vi "InAs-GaAs superlattice-111227a.vi"() -> ()   [LabVIEW 2011]
panel:
  out "step number  5":i32
  in  "Number of \nGrowth Steps 5":i32=10
  out "step number  4":i32
  in  "Number of \nGrowth Steps 4":i32=10
  out "step number  3":i32
  in  "Number of \nGrowth Steps 3":i32=10
  out "step number  2":i32
  in  "Number of \nGrowth Steps 2":i32=10
  in  "Ga Flow 1":dbl=5.49
  in  "Indium Flow":dbl=45.0
  in  "Number of \nGrowth Steps":i32=10
  out "step number":i32
  in  "As_Gas Flow":dbl=3.4
  in  "Manifold H2 Flow":dbl=730.0
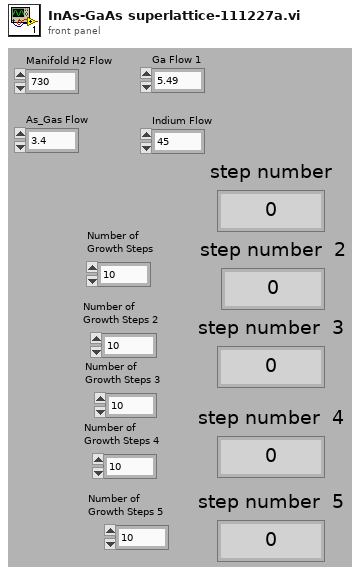
[diagram p1: front panel]
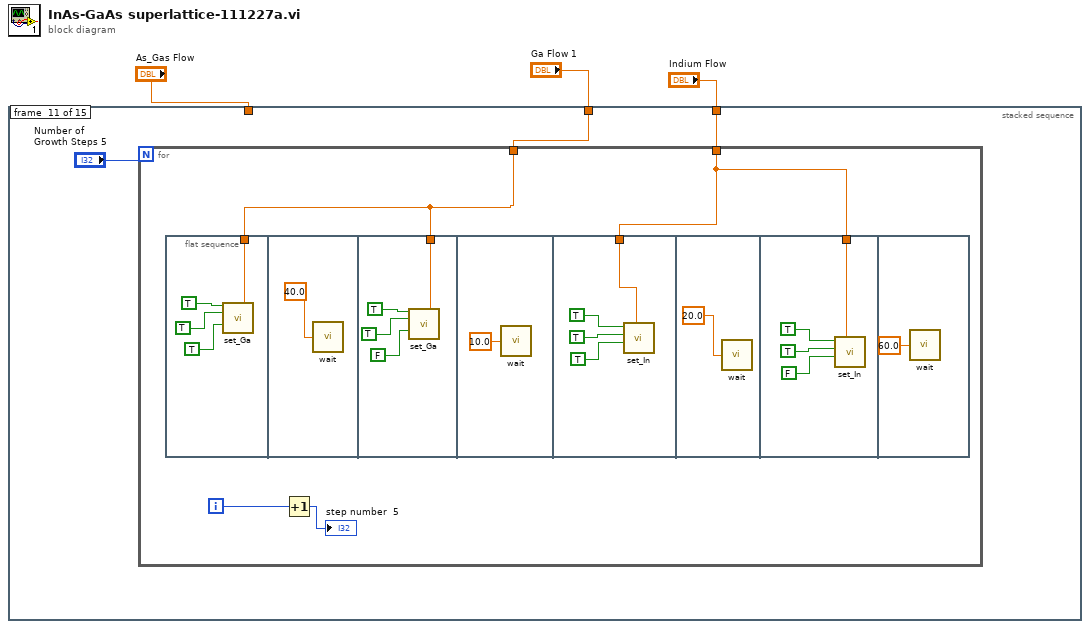
[diagram p0: block diagram]
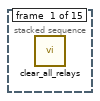
[diagram p2: hidden frame]
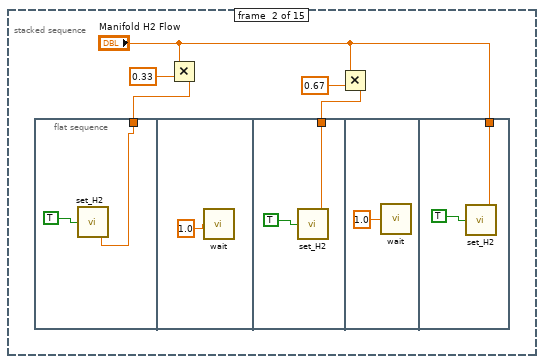
[diagram p3: hidden frame]
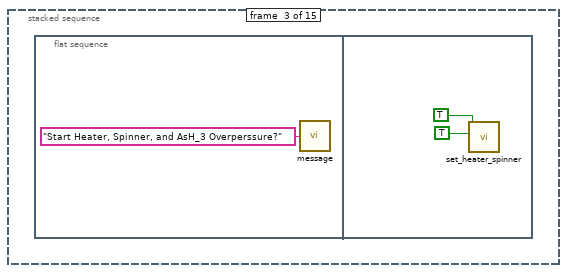
[diagram p4: hidden frame]
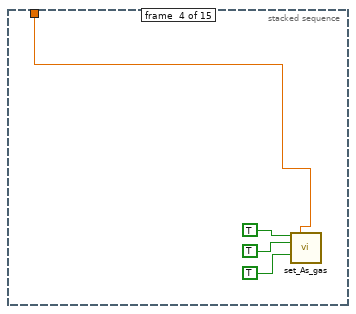
[diagram p5: hidden frame]
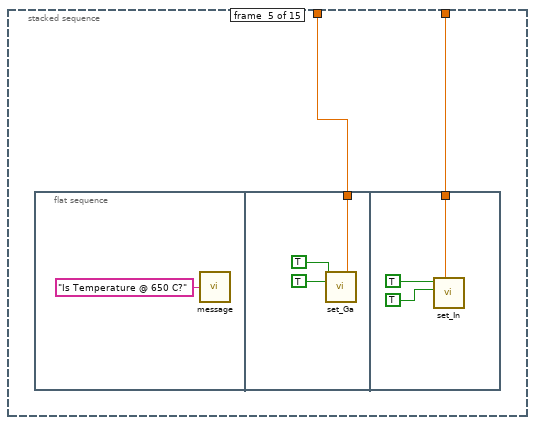
[diagram p6: hidden frame]
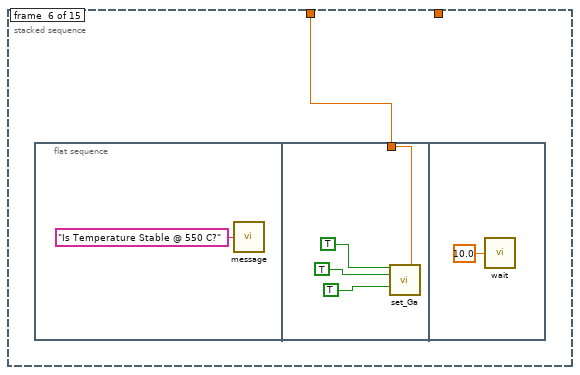
[diagram p7: hidden frame]
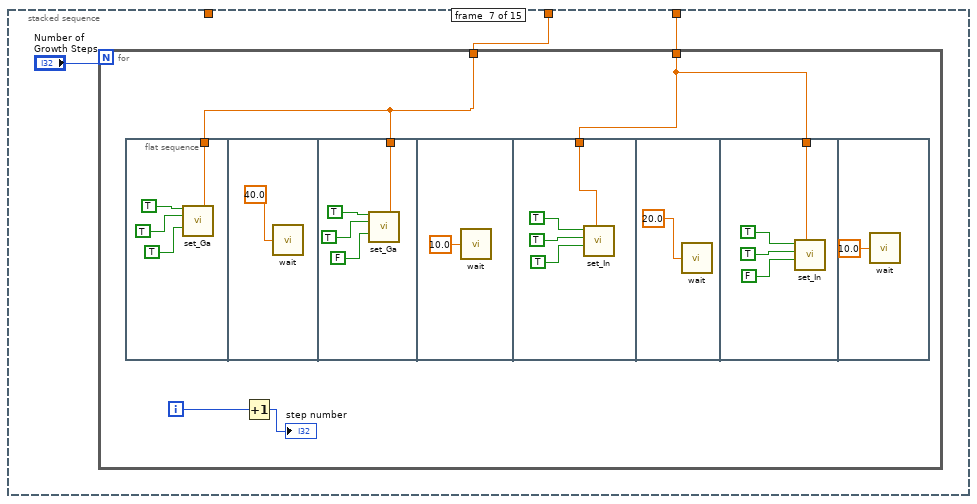
[diagram p8: hidden frame]
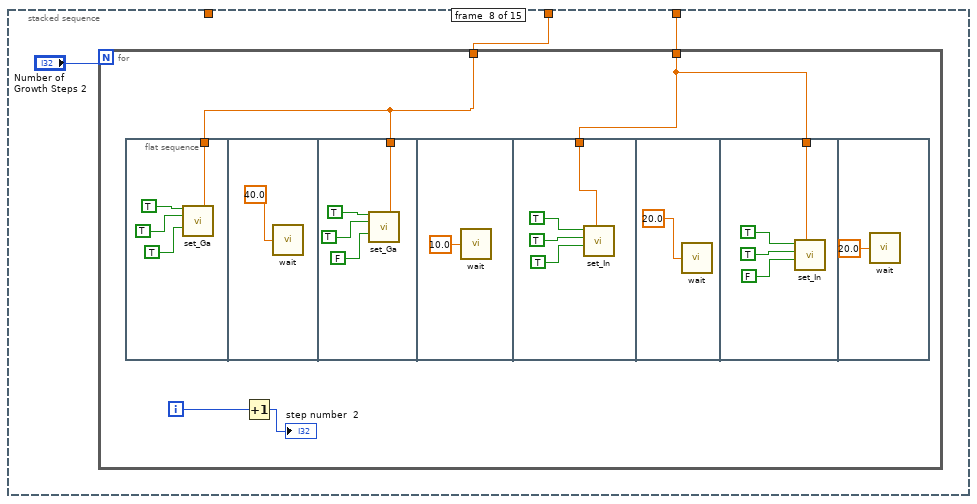
[diagram p9: hidden frame]
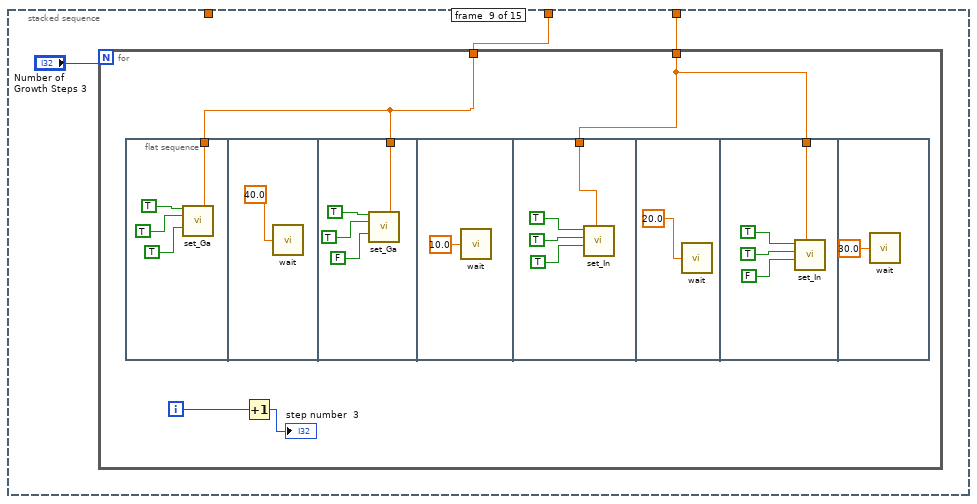
[diagram p10: hidden frame]
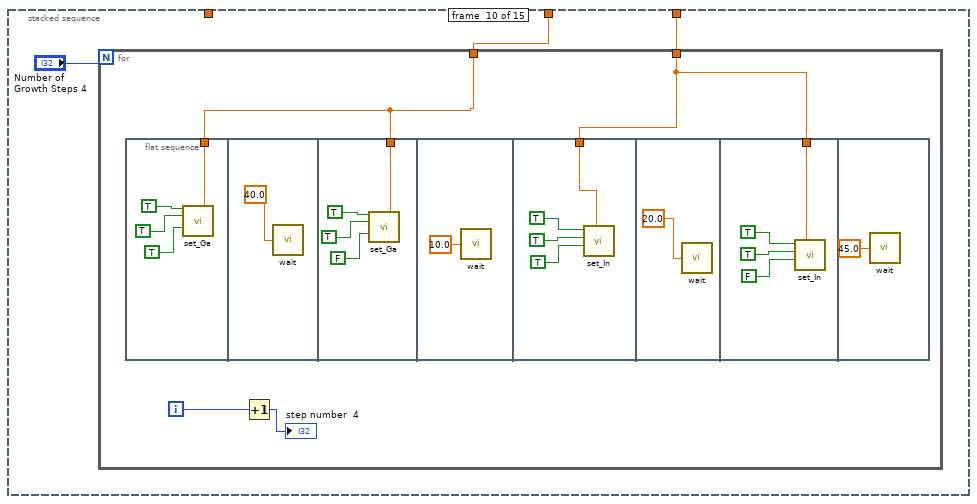
[diagram p11: hidden frame]
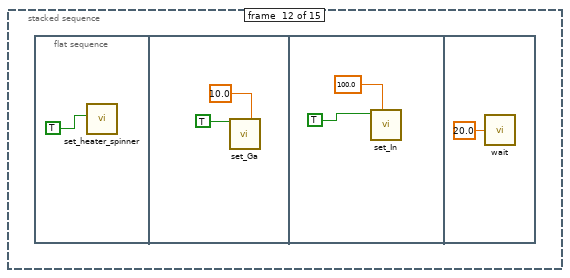
[diagram p12: hidden frame]
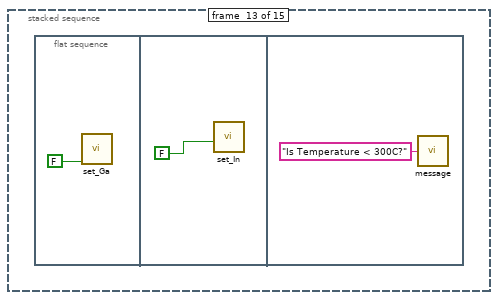
[diagram p13: hidden frame]
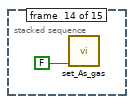
[diagram p14: hidden frame]
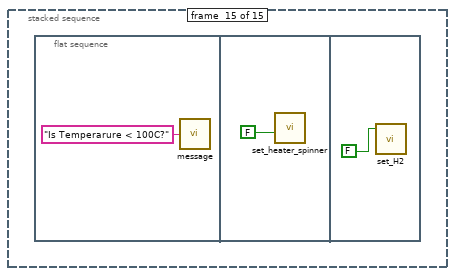
[diagram p15: hidden frame]
diagram:
  n1 = stacked-sequence {
    tunnel: "Ga Flow 1" -> [_ _ _ _ w25 w33 w41 w68 w95 w122 w149 _ _ _ _]
    tunnel: "As_Gas Flow" -> [_ _ _ w20 _ _ _ _ _ _ _ _ _ _ _]
    tunnel: "Indium Flow" -> [_ _ _ _ w24 _ w40 w67 w94 w121 w148 _ _ _ _]
    frame #0 {
      n2 = call "clear_all_relays.vi"() -> ()  [unwired: 2 out]
    }
    frame #1 {
      n3 = flat-sequence {
        tunnel: w8 -> [w9]
        tunnel: w6 -> [w12]
        tunnel: "Manifold H2 Flow" -> [w15]
        frame #0 {
          n4 = call "set_H2.vi"("Manifold H2 Flow"=w9, "H2 Active"=TRUE) -> ()  [unwired: 2 in, 2 out]
        }
        frame #1 {
          n5 = call "wait.vi"("Wait (s)"=1.0) -> ()  [unwired: 1 out]
        }
        frame #2 {
          n6 = call "set_H2.vi"("Manifold H2 Flow"=w12, "H2 Active"=TRUE) -> ()  [unwired: 2 in, 2 out]
        }
        frame #3 {
          n7 = call "wait.vi"("Wait (s)"=1.0) -> ()  [unwired: 1 out]
        }
        frame #4 {
          n8 = call "set_H2.vi"("Manifold H2 Flow"=w15, "H2 Active"=TRUE) -> ()  [unwired: 2 in, 2 out]
        }
      }
      n9 = Multiply(x="Manifold H2 Flow", y=0.33) -> (x*y=w8:dbl)
      n10 = Multiply(x="Manifold H2 Flow", y=0.67) -> (x*y=w6:dbl)
    }
    frame #2 {
      n11 = flat-sequence {
        frame #0 {
          n12 = call "message.vi"("message"="Start Heater, Spinner, and AsH_3 Overperssure?") -> ()
        }
        frame #1 {
          n13 = call "set_heater_spinner.vi"("Spinner"=TRUE, "Heater"=TRUE) -> ()  [unwired: 1 in, 7 out]
        }
      }
    }
    frame #3 {
      n14 = call "set_As_gas.vi"("As_Gas Active"=TRUE, "As_Gas Flow"=w20, "As_Gas In"=TRUE, "As_Gas Run"=TRUE) -> ()  [unwired: 2 in, 10 out]
    }
    frame #4 {
      n15 = flat-sequence {
        tunnel: w25 -> [w27]
        tunnel: w24 -> [w30]
        frame #0 {
          n16 = call "message.vi"("message"="Is Temperature @ 650 C?") -> ()
        }
        frame #1 {
          n17 = call "set_Ga.vi"("Ga Active"=TRUE, "Ga Flow 1"=w27, "Ga Bubbler"=TRUE) -> ()  [unwired: 5 in, 8 out]
        }
        frame #2 {
          n18 = call "set_In.vi"("Indium Flow"=w30, "In Bubbler"=TRUE ("Ga Bubbler"), "In Active"=TRUE ("Ga Active")) -> ()  [unwired: 2 in, 5 out]
        }
      }
    }
    frame #5 {
      n19 = flat-sequence {
        tunnel: w33 -> [w35]
        frame #0 {
          n20 = call "message.vi"("message"="Is Temperature Stable @ 550 C?") -> ()
        }
        frame #1 {
          n21 = call "set_Ga.vi"("Ga Active"=TRUE ("P_Gas Active"), "Ga Flow 1"=w35, "Ga Bubbler"=TRUE ("P_Gas In"), "Ga Run"=TRUE ("P_Gas Run")) -> ()  [unwired: 4 in, 8 out]
        }
        frame #2 {
          n22 = call "wait.vi"("Wait (s)"=10.0) -> ()  [unwired: 1 out]
        }
      }
    }
    frame #6 {
      n23 = for {
        N: "Number of \nGrowth Steps" -> [_]
        tunnel: w41 -> [w44]
        tunnel: w40 -> [w43]
        i -> [w45]
        n24 = flat-sequence {
          tunnel: w44 -> [w47]
          tunnel: w44 -> [w52]
          tunnel: w43 -> [w57]
          tunnel: w43 -> [w62]
          frame #0 {
            n25 = call "set_Ga.vi"("Ga Active"=TRUE ("P_Gas Active"), "Ga Flow 1"=w47, "Ga Bubbler"=TRUE ("P_Gas In"), "Ga Run"=TRUE ("P_Gas Run")) -> ()  [unwired: 4 in, 8 out]
          }
          frame #1 {
            n26 = call "wait.vi"("Wait (s)"=40.0) -> ()  [unwired: 1 out]
          }
          frame #2 {
            n27 = call "set_Ga.vi"("Ga Active"=TRUE ("P_Gas Active"), "Ga Flow 1"=w52, "Ga Bubbler"=TRUE ("P_Gas In"), "Ga Run"=FALSE ("P_Gas Run")) -> ()  [unwired: 4 in, 8 out]
          }
          frame #3 {
            n28 = call "wait.vi"("Wait (s)"=10.0) -> ()  [unwired: 1 out]
          }
          frame #4 {
            n29 = call "set_In.vi"("Indium Flow"=w57, "In Run"=TRUE ("P_Gas Run"), "In Bubbler"=TRUE ("P_Gas In"), "In Active"=TRUE ("P_Gas Active")) -> ()  [unwired: 1 in, 5 out]
          }
          frame #5 {
            n30 = call "wait.vi"("Wait (s)"=20.0) -> ()  [unwired: 1 out]
          }
          frame #6 {
            n31 = call "set_In.vi"("Indium Flow"=w62, "In Run"=FALSE ("P_Gas Run"), "In Bubbler"=TRUE ("P_Gas In"), "In Active"=TRUE ("P_Gas Active")) -> ()  [unwired: 1 in, 5 out]
          }
          frame #7 {
            n32 = call "wait.vi"("Wait (s)"=10.0) -> ()  [unwired: 1 out]
          }
        }
        n33 = Increment(x=w45) -> (x+1=→"step number":i32)
      }
    }
    frame #7 {
      n34 = for {
        N: "Number of \nGrowth Steps 2" -> [_]
        tunnel: w68 -> [w71]
        tunnel: w67 -> [w70]
        i -> [w72]
        n35 = flat-sequence {
          tunnel: w71 -> [w74]
          tunnel: w71 -> [w79]
          tunnel: w70 -> [w84]
          tunnel: w70 -> [w89]
          frame #0 {
            n36 = call "set_Ga.vi"("Ga Active"=TRUE ("P_Gas Active"), "Ga Flow 1"=w74, "Ga Bubbler"=TRUE ("P_Gas In"), "Ga Run"=TRUE ("P_Gas Run")) -> ()  [unwired: 4 in, 8 out]
          }
          frame #1 {
            n37 = call "wait.vi"("Wait (s)"=40.0) -> ()  [unwired: 1 out]
          }
          frame #2 {
            n38 = call "set_Ga.vi"("Ga Active"=TRUE ("P_Gas Active"), "Ga Flow 1"=w79, "Ga Bubbler"=TRUE ("P_Gas In"), "Ga Run"=FALSE ("P_Gas Run")) -> ()  [unwired: 4 in, 8 out]
          }
          frame #3 {
            n39 = call "wait.vi"("Wait (s)"=10.0) -> ()  [unwired: 1 out]
          }
          frame #4 {
            n40 = call "set_In.vi"("Indium Flow"=w84, "In Run"=TRUE ("P_Gas Run"), "In Bubbler"=TRUE ("P_Gas In"), "In Active"=TRUE ("P_Gas Active")) -> ()  [unwired: 1 in, 5 out]
          }
          frame #5 {
            n41 = call "wait.vi"("Wait (s)"=20.0) -> ()  [unwired: 1 out]
          }
          frame #6 {
            n42 = call "set_In.vi"("Indium Flow"=w89, "In Run"=FALSE ("P_Gas Run"), "In Bubbler"=TRUE ("P_Gas In"), "In Active"=TRUE ("P_Gas Active")) -> ()  [unwired: 1 in, 5 out]
          }
          frame #7 {
            n43 = call "wait.vi"("Wait (s)"=20.0) -> ()  [unwired: 1 out]
          }
        }
        n44 = Increment(x=w72) -> (x+1=→"step number  2":i32)
      }
    }
    frame #8 {
      n45 = for {
        N: "Number of \nGrowth Steps 3" -> [_]
        tunnel: w95 -> [w98]
        tunnel: w94 -> [w97]
        i -> [w99]
        n46 = flat-sequence {
          tunnel: w98 -> [w101]
          tunnel: w98 -> [w106]
          tunnel: w97 -> [w111]
          tunnel: w97 -> [w116]
          frame #0 {
            n47 = call "set_Ga.vi"("Ga Active"=TRUE ("P_Gas Active"), "Ga Flow 1"=w101, "Ga Bubbler"=TRUE ("P_Gas In"), "Ga Run"=TRUE ("P_Gas Run")) -> ()  [unwired: 4 in, 8 out]
          }
          frame #1 {
            n48 = call "wait.vi"("Wait (s)"=40.0) -> ()  [unwired: 1 out]
          }
          frame #2 {
            n49 = call "set_Ga.vi"("Ga Active"=TRUE ("P_Gas Active"), "Ga Flow 1"=w106, "Ga Bubbler"=TRUE ("P_Gas In"), "Ga Run"=FALSE ("P_Gas Run")) -> ()  [unwired: 4 in, 8 out]
          }
          frame #3 {
            n50 = call "wait.vi"("Wait (s)"=10.0) -> ()  [unwired: 1 out]
          }
          frame #4 {
            n51 = call "set_In.vi"("Indium Flow"=w111, "In Run"=TRUE ("P_Gas Run"), "In Bubbler"=TRUE ("P_Gas In"), "In Active"=TRUE ("P_Gas Active")) -> ()  [unwired: 1 in, 5 out]
          }
          frame #5 {
            n52 = call "wait.vi"("Wait (s)"=20.0) -> ()  [unwired: 1 out]
          }
          frame #6 {
            n53 = call "set_In.vi"("Indium Flow"=w116, "In Run"=FALSE ("P_Gas Run"), "In Bubbler"=TRUE ("P_Gas In"), "In Active"=TRUE ("P_Gas Active")) -> ()  [unwired: 1 in, 5 out]
          }
          frame #7 {
            n54 = call "wait.vi"("Wait (s)"=30.0) -> ()  [unwired: 1 out]
          }
        }
        n55 = Increment(x=w99) -> (x+1=→"step number  3":i32)
      }
    }
    frame #9 {
      n56 = for {
        N: "Number of \nGrowth Steps 4" -> [_]
        tunnel: w122 -> [w125]
        tunnel: w121 -> [w124]
        i -> [w126]
        n57 = flat-sequence {
          tunnel: w125 -> [w128]
          tunnel: w125 -> [w133]
          tunnel: w124 -> [w138]
          tunnel: w124 -> [w143]
          frame #0 {
            n58 = call "set_Ga.vi"("Ga Active"=TRUE ("P_Gas Active"), "Ga Flow 1"=w128, "Ga Bubbler"=TRUE ("P_Gas In"), "Ga Run"=TRUE ("P_Gas Run")) -> ()  [unwired: 4 in, 8 out]
          }
          frame #1 {
            n59 = call "wait.vi"("Wait (s)"=40.0) -> ()  [unwired: 1 out]
          }
          frame #2 {
            n60 = call "set_Ga.vi"("Ga Active"=TRUE ("P_Gas Active"), "Ga Flow 1"=w133, "Ga Bubbler"=TRUE ("P_Gas In"), "Ga Run"=FALSE ("P_Gas Run")) -> ()  [unwired: 4 in, 8 out]
          }
          frame #3 {
            n61 = call "wait.vi"("Wait (s)"=10.0) -> ()  [unwired: 1 out]
          }
          frame #4 {
            n62 = call "set_In.vi"("Indium Flow"=w138, "In Run"=TRUE ("P_Gas Run"), "In Bubbler"=TRUE ("P_Gas In"), "In Active"=TRUE ("P_Gas Active")) -> ()  [unwired: 1 in, 5 out]
          }
          frame #5 {
            n63 = call "wait.vi"("Wait (s)"=20.0) -> ()  [unwired: 1 out]
          }
          frame #6 {
            n64 = call "set_In.vi"("Indium Flow"=w143, "In Run"=FALSE ("P_Gas Run"), "In Bubbler"=TRUE ("P_Gas In"), "In Active"=TRUE ("P_Gas Active")) -> ()  [unwired: 1 in, 5 out]
          }
          frame #7 {
            n65 = call "wait.vi"("Wait (s)"=45.0) -> ()  [unwired: 1 out]
          }
        }
        n66 = Increment(x=w126) -> (x+1=→"step number  4":i32)
      }
    }
    frame #10 {
      n67 = for {
        N: "Number of \nGrowth Steps 5" -> [_]
        tunnel: w149 -> [w152]
        tunnel: w148 -> [w151]
        i -> [w153]
        n68 = flat-sequence {
          tunnel: w152 -> [w155]
          tunnel: w152 -> [w160]
          tunnel: w151 -> [w165]
          tunnel: w151 -> [w170]
          frame #0 {
            n69 = call "set_Ga.vi"("Ga Active"=TRUE ("P_Gas Active"), "Ga Flow 1"=w155, "Ga Bubbler"=TRUE ("P_Gas In"), "Ga Run"=TRUE ("P_Gas Run")) -> ()  [unwired: 4 in, 8 out]
          }
          frame #1 {
            n70 = call "wait.vi"("Wait (s)"=40.0) -> ()  [unwired: 1 out]
          }
          frame #2 {
            n71 = call "set_Ga.vi"("Ga Active"=TRUE ("P_Gas Active"), "Ga Flow 1"=w160, "Ga Bubbler"=TRUE ("P_Gas In"), "Ga Run"=FALSE ("P_Gas Run")) -> ()  [unwired: 4 in, 8 out]
          }
          frame #3 {
            n72 = call "wait.vi"("Wait (s)"=10.0) -> ()  [unwired: 1 out]
          }
          frame #4 {
            n73 = call "set_In.vi"("Indium Flow"=w165, "In Run"=TRUE ("P_Gas Run"), "In Bubbler"=TRUE ("P_Gas In"), "In Active"=TRUE ("P_Gas Active")) -> ()  [unwired: 1 in, 5 out]
          }
          frame #5 {
            n74 = call "wait.vi"("Wait (s)"=20.0) -> ()  [unwired: 1 out]
          }
          frame #6 {
            n75 = call "set_In.vi"("Indium Flow"=w170, "In Run"=FALSE ("P_Gas Run"), "In Bubbler"=TRUE ("P_Gas In"), "In Active"=TRUE ("P_Gas Active")) -> ()  [unwired: 1 in, 5 out]
          }
          frame #7 {
            n76 = call "wait.vi"("Wait (s)"=60.0) -> ()  [unwired: 1 out]
          }
        }
        n77 = Increment(x=w153) -> (x+1=→"step number  5":i32)
      }
    }
    frame #11 {
      n78 = flat-sequence {
        frame #0 {
          n79 = call "set_heater_spinner.vi"("Spinner"=TRUE ("Ga Active")) -> ()  [unwired: 2 in, 7 out]
        }
        frame #1 {
          n80 = call "set_Ga.vi"("Ga Active"=TRUE, "Ga Flow 1"=10.0) -> ()  [unwired: 6 in, 8 out]
        }
        frame #2 {
          n81 = call "set_In.vi"("Indium Flow"=100.0 ("Aluminum Flow"), "In Active"=TRUE ("Ga Active")) -> ()  [unwired: 3 in, 5 out]
        }
        frame #3 {
          n82 = call "wait.vi"("Wait (s)"=20.0) -> ()  [unwired: 1 out]
        }
      }
    }
    frame #12 {
      n83 = flat-sequence {
        frame #0 {
          n84 = call "set_Ga.vi"("Ga Remote"=FALSE) -> ()  [unwired: 7 in, 8 out]
        }
        frame #1 {
          n85 = call "set_In.vi"("In Run"=FALSE ("Ga Remote")) -> ()  [unwired: 4 in, 5 out]
        }
        frame #2 {
          n86 = call "message.vi"("message"="Is Temperature < 300C?") -> ()
        }
      }
    }
    frame #13 {
      n87 = call "set_As_gas.vi"("As_Gas Remote"=FALSE) -> ()  [unwired: 5 in, 10 out]
    }
    frame #14 {
      n88 = flat-sequence {
        frame #0 {
          n89 = call "message.vi"("message"="Is Temperarure < 100C?") -> ()
        }
        frame #1 {
          n90 = call "set_heater_spinner.vi"("Heater/Spinner Remote"=FALSE) -> ()  [unwired: 2 in, 7 out]
        }
        frame #2 {
          n91 = call "set_H2.vi"("H2N2 Remote"=FALSE) -> ()  [unwired: 3 in, 2 out]
        }
      }
    }
  }
